vi "UpdateDashboard.vi"   [LabVIEW 2010]
uses:
  7.0-Global.vi
types:
  T1 = cluster{"Speed":dbl, "Heading":dbl, "Battery":dbl, "Time":dbl}
  T2 = typedef "MainIndicators.ctl" = cluster{"Where?":bool, "What?":bool, "4.2-Where Am I? Sensor":T3, "4.3-What's Around Me? Sensor":T6, "5.3.1 MissionTimeAuto":dbl, "5.4 Clean How Am I? Sensor":T8, "How?":bool}
  T3 = typedef "4.2-Where Sensor Typedef.ctl" = cluster{"4.2.2- Current GPS Data":T4, "4.2.1-VectorNav Data":T5, "4.2.1-VectorNav Status":string}
  T4 = typedef "Current GPS Data.ctl" = cluster{"Lattitude (dd.mmmmmm)":ext, "Longitude (dd.mmmmmm)":ext, "EST Time":timestamp}
  T5 = typedef "3.2.1-VectorNav Data.ctl" = cluster{"Yaw":dbl, "Pitch":dbl, "Roll":dbl}
  T6 = typedef "4.3-What Sensor Typedef.ctl" = cluster{"LIDAR Data":T7}
  T7 = typedef "3.3.1-LIDAR Data Typedef.ctl" = cluster{"Angle array":dbl[], "Magnitude array ":dbl[]}
  T8 = typedef "5.4-Clean How Sensor Typedef.ctl" = cluster{"Motor Speed Integer":i32, "Drive Position Integer":i32, "Lidar Position Integer":i32, "Lidar Motor Position Integer":i32, "Steering Position Integer":i32, "Battery Voltage Fxp":dbl, "Drive Encoder Cable Check":bool, "Lidar Drive Encoder Cable Check":bool, "Steer Encoder Cable Check":bool, "Lidar Pos Encoder Cable Check":bool, "Mod Buttons & Blinky Cable Check":bool, "Lidar Data Cable Check":bool, "Drive Motor Cable Check":bool, "Vector Nav Cable Check":bool, "Lidar Drive Cable Check":bool, "Steer Drive Cable Check":bool, "Reverse?":bool, "2.1  Steering Control Voltage":dbl, "2.1 Drive Control Voltage":dbl, "2.1  Lidar Control Voltage":dbl, "2.5.7 A*B":dbl, "2.1  Steering PID Output":dbl, "2.1 Drive PID Output":dbl, "2.1  Lidar PID Output":dbl, "2.1.1 Drive Error":dbl, "2.1.1 Drive Error I":dbl, "2.1.1 Drive Error D":dbl, "2.1.2 Steering Error":dbl, "2.1.2 Steering Error I":dbl, "2.1.2 Steering Error D":dbl, "2.1.3 Lidar Error":dbl, "2.1.3 Lidar Error I":dbl, "2.1.3 Lidar Error D":dbl, "VectorNav Ack Query":bool, "VectorNav Read Byte":u8, "VectorNav Read Status":enum16{"Waiting", "Reading", "Done"}}
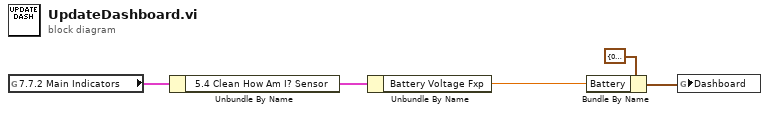
[diagram p0: block diagram]
diagram:
  n1 = global read "7.0-Global.vi" "7.7.2 Main Indicators"() -> (w5:T2)
  n2 = Unbundle By Name(w5) -> ("5.4 Clean How Am I? Sensor"=w4:T8)
  n3 = Unbundle By Name(w4) -> ("Battery Voltage Fxp"=w1:dbl)
  n4 = Bundle By Name(cluster=T1 {"Speed"=0.0, "Heading"=0.0, "Battery"=0.0, "Time"=0.0} ("Cluster"), "Battery"=w1) -> (w3:T1)
  n5 = global write "7.0-Global.vi" "Dashboard"(w3) -> ()
